vi "EuniceF_Project4.vi"() -> ()   [LabVIEW 2025]
panel:
  out "HIGH":bool
  out "LOW":bool
  out "Temperature, C":dbl(graph)
  out "Thermometer, C":dbl(slide) scale=0.0..100.0
  in  "stop":bool
  out "AtoD":i16 format="%x"
  out "R,kOhms":dbl(slide) scale=0.0..30.0 scale format="%.2g"
  out "Vscc,V":dbl(slide) scale=0.0..6.0 scale format="%.3g"
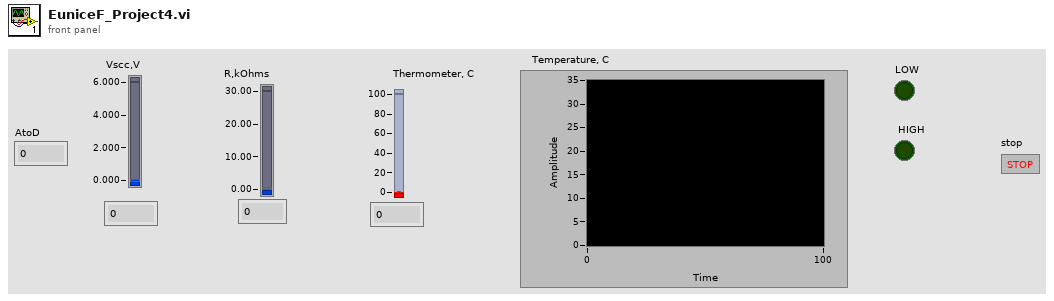
[diagram p1: front panel]
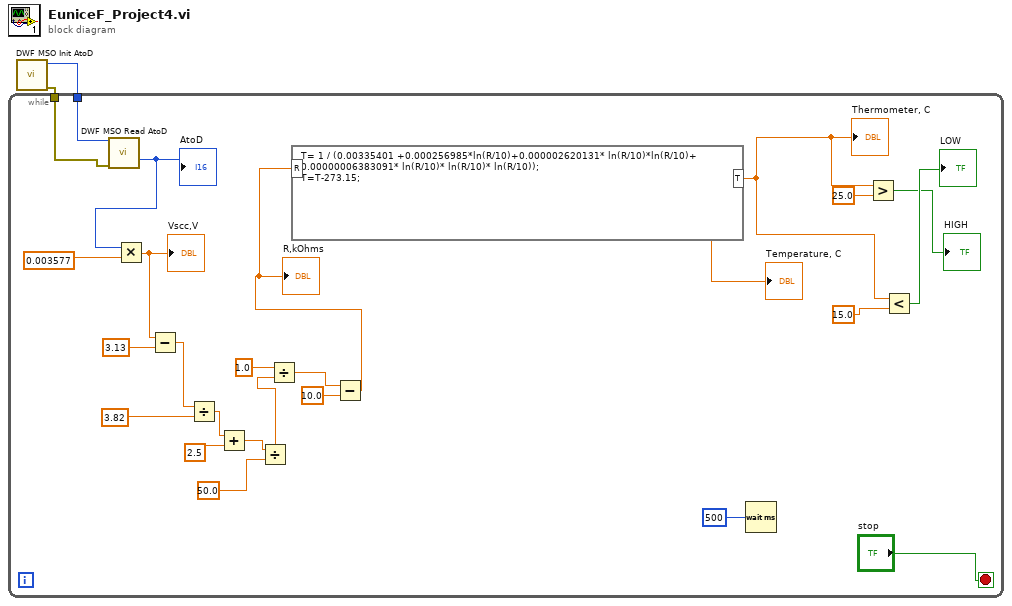
[diagram p0: block diagram]
diagram:
  n1 = call "DWF MSO Init AtoD.vi"() -> ("Error Out"=w1:errorcluster, "Instrument Handle Out"=w2:i32)  [unwired: 10 in]
  n2 = while {
    tunnel: w2 -> [w26]
    tunnel: w1 -> [w25]
    stop <- "stop" stop-if-true
    n3 = call "DWF MSO Read AtoD.vi"("Instrument Handle In AtoD"=w26, "Error In"=w25) -> ("AtoD"=w24:i16)  [unwired: 12 in, 1 out]
    "AtoD" <- w24
    n4 = Multiply(x=w24, y=0.003577) -> (x*y=w22:dbl)
    "Vscc,V" <- w22
    n5 = Subtract(x=w22, y=3.13) -> (x-y=w19:dbl)
    n6 = Divide(x=w19, y=3.82) -> (x/y=w18:dbl)
    n7 = Add(x=w18, y=2.5) -> (x+y=w16:dbl)
    n8 = Divide(x=w16, y=50.0) -> (x/y=w13:dbl)
    n9 = Divide(x=1.0, y=w13) -> (x/y=w12:dbl)
    n10 = Subtract(x=w12, y=10.0) -> (x-y=w8:dbl)
    "R,kOhms" <- w8
    n11 = formula code="T= 1 / (0.00335401 +0.000256985*ln(R/10)+0.000002620131* ln(R/10)*ln(R/10)+ 0.00000006383091* ln(R/10)* ln(R/10)* ln(R/10));\nT=T-273.15;"("R"=w8) -> ("T"=w5:dbl)
    "Thermometer, C" <- w5
    "Temperature, C" <- w5
    n12 = Wait (ms)(milliseconds to wait=u32 500) -> ()  [unwired: 1 out]
    n13 = Greater?(x=w5, y=25.0) -> (0:→"HIGH":bool)
    n14 = Less?(x=w5, y=15.0) -> (x < y?=→"LOW":bool)
  }
